vi "Close Comm Refs.vi"(8 "error in":errorcluster, 11 "Comm.lvclass":refnum<class "VeriStand Comm.lvclass">) -> (0 "error out":errorcluster)   [LabVIEW 2019, in "NI VeriStand Addon Network Comm.lvlib" / "VeriStand Comm.lvclass"]
uses:
  VeriStand Comm.lvclass
  VeriStand Comm.lvclass/VeriStand Comm.ctl
  <vilib>/NI/STM/Connection Manager/TCP/TCP Connection Method.ctl
  <vilib>/NI/STM/SubVIs/Generate STM Error.vi
  <vilib>/NI VeriStand/Custom Device Tools/Custom Device Utility Library/Custom Device Utility Library.lvlib
  <vilib>/NI/STM/NI STM.lvlib
  <vilib>/NI/AMC/AMC.lvlib
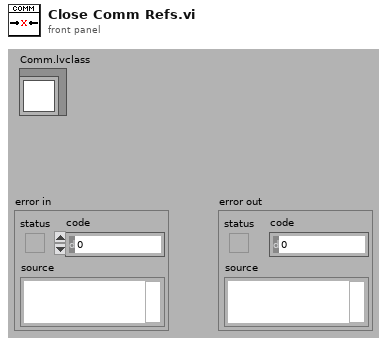
[diagram p1: front panel]
types:
  T1 = typedef "NI STM.lvlib/TCP Connection Method.ctl" = enum16{"Initialize", "Add Connection", "Set Properties", "Get Connection(s)", "Remove Connection", "Remove All Connections", "Get Connection Count"}
  T2 = typedef "AMC.lvlib/Message Queue.ctl" = refnum<queue>
  T3 = typedef "NI STM.lvlib/TCP Connection Manager Reference.ctl" = refnum<data-value>
  T4 = typedef "NI STM.lvlib/TCP Connection Info.ctl" = cluster{"connection ID":refnum<k5>, "meta data":T5[]}
  T5 = typedef "NI STM.lvlib/MetaDataElement.ctl" = string
  T6 = typedef "NI STM.lvlib/TCP Connection Properties.ctl" = cluster{"Name":string, "Address":string, "Custom":string}
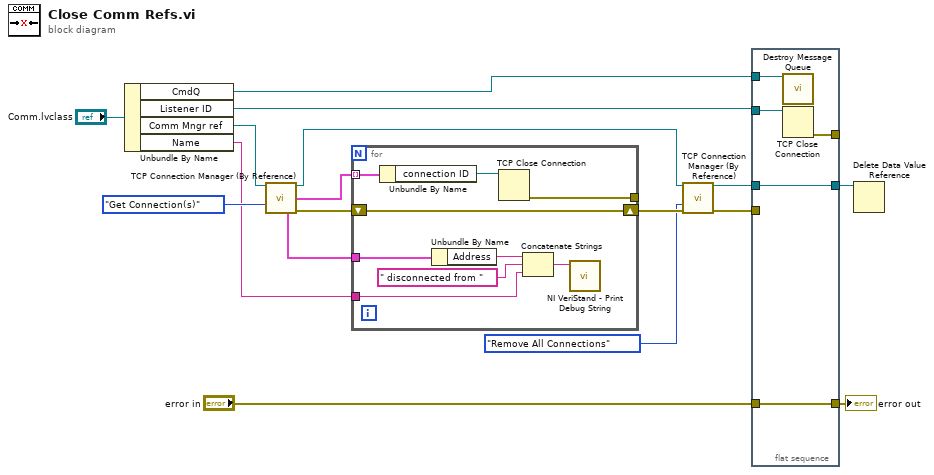
[diagram p0: block diagram]
diagram:
  n1 = Unbundle By Name("Comm.lvclass") -> ("CmdQ"=w1:T2, "Listener ID"=w5:refnum<k5>, "Comm Mngr ref"=w6:T3, "Name"=w2:string)
  n2 = call <vilib>:"TCP Connection Manager (By Reference).vi"("connection manager ref in"=w6, "method"=TCP_Connection_Method."Get Connection(s)") -> ("connection manager ref out"=w9:T3, "all connections"=w15:T4[], "properties out"=w8:T6, "error out"=w14:errorcluster)  [unwired: 7 in, 3 out]
  n3 = for {
    tunnel: w15 -> [w18] mode=indexing
    shift-right: [w24] -> w13
    shift-left: w14 -> [w24]
    tunnel: [w25] -> _
    tunnel: w2 -> [w20]
    tunnel: w8 -> [w19]
    n4 = Unbundle By Name(w18) -> ("connection ID"=w26:refnum<k5>)
    n5 = Unbundle By Name(w19) -> ("Address"=w21:string)
    n6 = TCP Close Connection(connection ID=w26) -> (error out=w25:errorcluster)  [unwired: 2 in, 1 out]
    n7 = Concatenate Strings(w21, " disconnected from " ("string"), w20) -> (w23:string)
    n8 = call <vilib>:"NI VeriStand - Print Debug String.vi"("Message"=w23) -> ()  [unwired: 10 in, 1 out]
  }
  n9 = call <vilib>:"TCP Connection Manager (By Reference).vi"("connection manager ref in"=w9, "method"=TCP_Connection_Method."Remove All Connections", "error in"=w13) -> ("connection manager ref out"=w11:T3, "error out"=w12:errorcluster)  [unwired: 6 in, 5 out]
  n10 = flat-sequence {
    tunnel: w5 -> [w31]
    tunnel: [w30] -> w17
    tunnel: w12 -> [_]
    tunnel: "error in" -> [w30]
    tunnel: [w29] -> _
    tunnel: w11 -> [w28]
    tunnel: [w28] -> w10
    tunnel: w1 -> [w27]
    frame #0 {
      n11 = call <vilib>:"Destroy Message Queue.vi"("message queue in"=w27) -> ()  [unwired: 12 in, 3 out]
      n12 = TCP Close Connection(connection ID=w31) -> (error out=w29:errorcluster)  [unwired: 2 in, 1 out]
    }
  }
  n13 = Delete Data Value Reference(data value reference=w10) -> ()  [unwired: 1 in, 2 out]
  "error out" <- w17
